vi "test_sound.vi"(10 "Sound File Path":path=path "C:/AGV/Config/sound/39150700348-point-mort-wav.wav", 11 "Device ID":u32) -> (3 "Sound Is Playing?":bool)   [LabVIEW 2019]
panel:
  in  "error":errorcluster caption="error in"
  out "error out":errorcluster
  out "웨이브폼 그래프":dbl[](graph)
  in  "Stop":bool
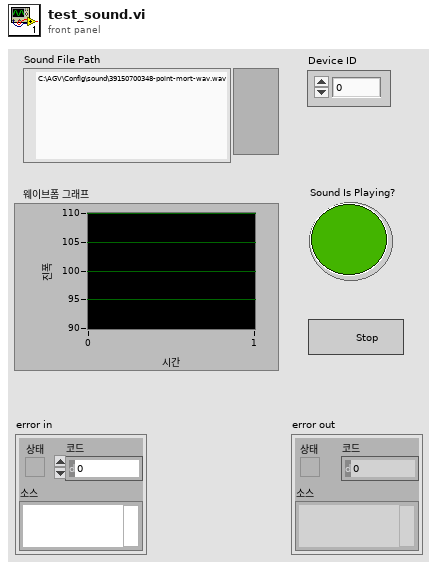
[diagram p1: front panel]
types:
  T1 = typedef "Sound Output Task ID.ctl" = u32
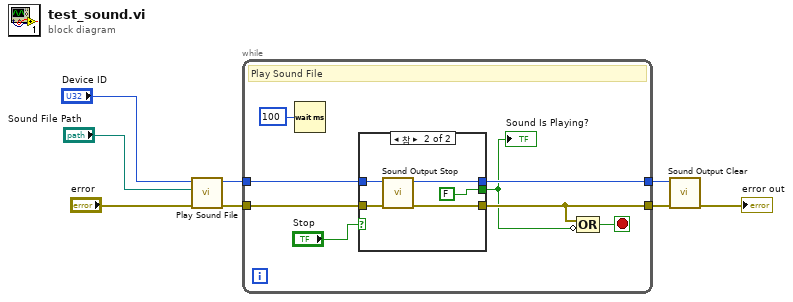
[diagram p0: block diagram]
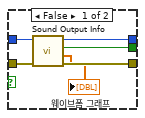
[diagram p2: hidden frame]
diagram:
  n1 = call <vilib>:"Play Sound File.vi"("error in (no error)"="error", "path"="Sound File Path", "device ID"="Device ID") -> ("error out"=w7:errorcluster, "task ID"=w8:T1)  [unwired: 7 in]
  n2 = while {
    tunnel: w8 -> [w10]
    tunnel: [w15] -> w5
    tunnel: w7 -> [w11]
    tunnel: [w14] -> w6
    stop <- w16 stop-if-true
    # "Play Sound File"
    n3 = Wait (ms)(milliseconds to wait=u32 100) -> ()  [unwired: 1 out]
    n4 = case shown="참" "Stop" {
      tunnel: w11 -> [w22 w26]
      tunnel: [w21 w24] -> w15
      tunnel: w10 -> [w20 w27]
      tunnel: [w19 w25] -> w14
      tunnel: [w18 FALSE] -> w13
      frame False {
        n5 = call <vilib>:"Sound Output Info.vi"("error in (no error)"=w22, "task ID"=w20) -> ("error out"=w19:errorcluster, "volume"=→"웨이브폼 그래프":dbl[], "is playing?"=w18:bool, "task ID out"=w21:T1)  [unwired: 6 in]
      }
      frame True {
        n6 = call <vilib>:"Sound Output Stop.vi"("error in (no error)"=w26, "task ID"=w27) -> ("error out"=w25:errorcluster, "task ID out"=w24:T1)  [unwired: 8 in]
      }
    }
    "Sound Is Playing?" <- w13
    n7 = Compound Arithmetic op=OR(w14, invert w13) -> (w16:bool)
  }
  n8 = call <vilib>:"Sound Output Clear.vi"("error in (no error)"=w6, "task ID"=w5) -> ("error out"=→"error out":errorcluster)  [unwired: 9 in]
